vi "mkCameraMain.vi"() -> ()   [LabVIEW 2011]
uses:
  BeadTracker2.llb/GlobalVariables.vi
  BeadTracker2.llb/CmdEnum_CameraIn.ctl
  BeadTracker2.llb/CmdData_GrabParams.ctl
  BeadTracker2.llb/CmdData_NewFrame.ctl
  BeadTracker2.llb/CmdEnum_CameraFrameType.ctl
  <vilib>/vision/Image Controls.llb/IMAQ Image.ctl
  qtrk/QTrk.llb/QTrkInstance.ctl
  CameraConfig.ctl
  CameraInterface.llb/CameraInterface.ctl
  BeadTracker2.llb/GenericCameraConfigType.ctl
panel:
  in  "Test vi ref interface":bool
  in  "Camera interface":T1
  in  "Config dialog":bool
  in  "Set QTrk dll":bool
  in  "Stop":bool
  in  "Tracking test":bool
  out "# elements in Camera In":i32
  in  "EndGrab":bool
  in  "GrabIdle":bool
  in  "Init":bool
  out "Have IMAQ Session?":bool
  in  "IMAQ Session":refnum<k11>
  out "Debug Indicator:\nCurrent grab state":T2
  in  "Camera msg type":T2
  in  "Send camera msg":bool
  in  "Camera settings":T3={"Gain [1-4]"=500.0, "Offset"=2, "Mode"=75, "ROIs"=[], "ROI Size"={"X"=0, "Y"=0}, "Number of buffers"=40, "Use hardware multiple-ROI?"=TRUE, "GenericCameraConfig"={"Framerate (Hz)"=1280, "Exposure time (us)"=1024, "Image size"={"Width"=1280, "Height"=1024}}}
  # "us"
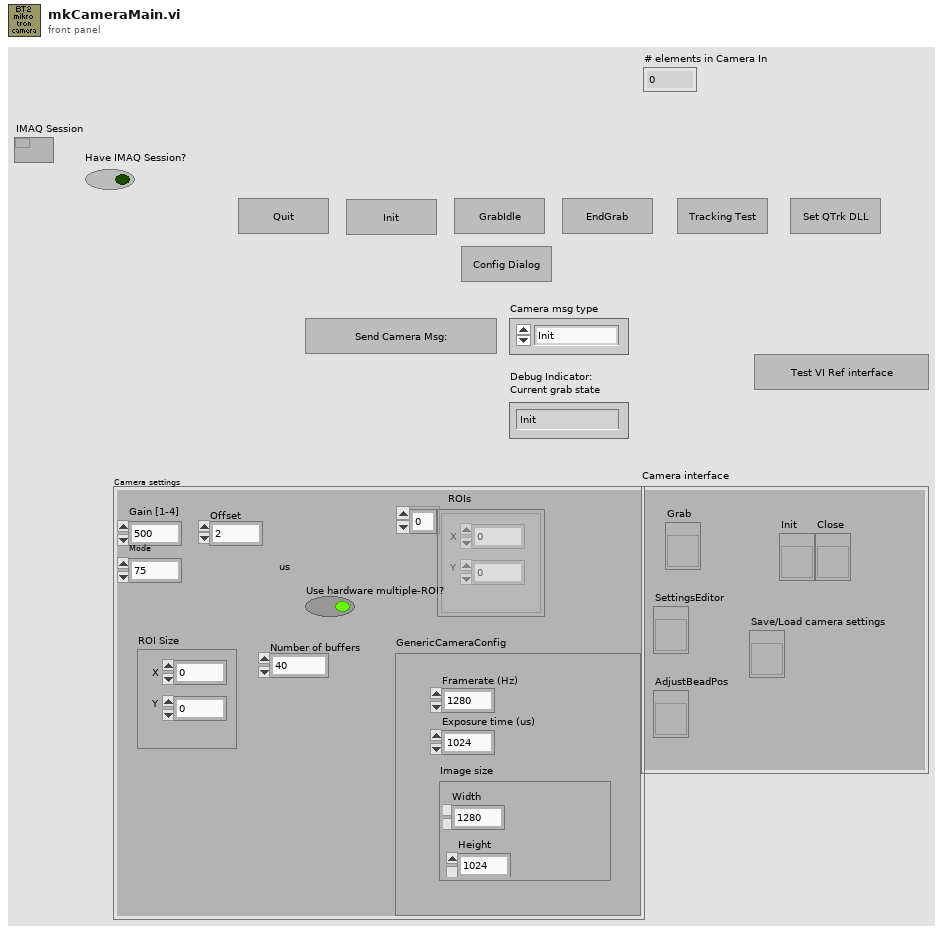
[diagram p1: front panel]
types:
  T1 = typedef "CameraInterface.ctl" = cluster{"SettingsEditor":refnum<vi>, "AdjustBeadPos":refnum<vi>, "Save/Load camera settings":refnum<vi>, "Init":refnum<vi>, "Close":refnum<vi>, "Grab":refnum<vi>}
  T2 = typedef "CmdEnum_CameraIn.ctl" = enum32{"Init", "Close", "ShowSettingsDialog", "EndGrab", "GrabZLUT", "GrabToTracker", "GrabToQueue", "AdjustROIs"}
  T3 = typedef "CameraConfig.ctl" = cluster{"Gain [1-4]":sgl, "Offset":i16, "Mode":i16, "ROIs":cluster{"X":i32, "Y":i32}[], "ROI Size":cluster{"X":i32, "Y":i32}, "Number of buffers":i32, "Use hardware multiple-ROI?":bool, "GenericCameraConfig":T4}
  T4 = typedef "GenericCameraConfigType.ctl" = cluster{"Framerate (Hz)":i32, "Exposure time (us)":i32, "Image size":cluster{"Width":i32, "Height":i32}}
  T5 = typedef "MeasureConfigType.ctl" = cluster{"Bead locations":cluster{"X":i32, "Y":i32}[], "ROI":i32, "Experiment base path":path, "Image output subdir":string, "Output mode":T6, "Traces output subdir":string, "QTrk Settings":T7, "Tracking Config":T8, "Experiment Name":string, "Program":T11, "ZLUT":sgl[][][], "Camera settings":T4, "Experiment Script":string, "Max frames in memory":i32, "Save traces as binary":bool, "Pixel Calibration Gain Image":string, "Pixel Calibration Offset Image":string, "Use pixel calibration images":bool}
  T6 = typedef "MeasureConfigOutputMode.ctl" = enum16{"None", "Track", "SaveImages"}
  T7 = typedef "QTrkSettings.ctl" = cluster{"Image width":i32, "Image height":i32, "Number of threads (CPU based)":i32, "CUDA Device":i32, "COM Background correction factor":sgl, "ZLUT MinRadius":sgl, "ZLUT Radial Coverage":sgl, "ZLUT Angular Coverage":sgl, "ZLUT ROI Coverage":sgl, "QI Iterations":i32, "QI MinRadius":sgl, "QI Radial Coverage":sgl, "QI Angular Coverage":sgl, "QI ROI Coverage":sgl, "QI Angular Step \nIteration Factor":sgl, "XCOR Profile Length":i32, "XCOR Profile Width":i32, "XCOR Iterations":i32, "Gaussian 2D Fit Iterations":i32, "Gaussian 2D Sigma (pixels)":sgl}
  T8 = typedef "TrackingConfigType.ctl" = cluster{"Number of steps":i32, "ZLUT stepsize (um)":sgl, "Z correction factor":sgl, "Start piezo Z (um)":sgl, "Pixel size (nm)":sgl, "2D Localization Type":T9, "Z Command (None)":T10}
  T9 = typedef "QTrkLocalizationType.ctl" = enum16{"Center-of-Mass", "1D Cross-Correlation", "Quadrant Interpolation", "Gaussian 2D MLE"}
  T10 = typedef "QTrkZCommandType.ctl" = enum16{"Nothing", "ComputeZ", "BuildRadialZLUT", "BuildImageZLUT", "RadialZLUT+ImageZLUT"}
  T11 = typedef "ExperimentProgramType.ctl" = cluster{"Commands":T12[], "Motor Axis accuracy conditions":T15, "Axis flags":T17}
  T12 = typedef "ExProgCommandType.ctl" = cluster{"cmd":T13, "axis":T14, "value/pos":dbl, "speed":dbl, "name":string}
  T13 = typedef "ExProgCommandEnumType.ctl" = enum16{"wait", "move", "acquire", "idle", "rmove", "when", "section", "stop"}
  T14 = typedef "MotorAxisEnum.ctl" = enum16{"no axis", "magrot", "magpos", "px", "py", "pz", "camx", "camy"}
  T15 = typedef "MotorPosType.ctl" = cluster{"Magnet Z":dbl, "Magnet rotation":dbl, "Camera":T16, "Piezo XY":T16, "Piezo Z":dbl}
  T16 = typedef "XYf.ctl" = cluster{"X":sgl, "Y":sgl}
  T17 = typedef "MotorPosFlagsType.ctl" = cluster{"Magnet Z":bool, "Magnet rotation":bool, "Camera":cluster{"X":bool, "Y":bool}, "Piezo XY":cluster{"X":bool, "Y":bool}, "Piezo Z":bool}
  T18 = typedef "QueueListType.ctl" = cluster{"Motor In":refnum<queue>, "User Interface Image View":refnum<queue>, "User Interface Camera Control":refnum<queue>, "User Interface Event Notifier":refnum<notifier>, "Initialized?":bool}
  T19 = typedef "CmdData_GrabParams.ctl" = cluster{"QTrk Instance":T20, "Output Queue":refnum<queue>}
  T20 = typedef "QTrkInstance.ctl" = cluster{"QTrk Pointer":u64}
  T21 = typedef "CmdData_NewFrame.ctl" = cluster{"Buffer Image":T22, "Frame #":i32, "Hardware ROI Index":i32, "Timestamp":dbl, "Type":T23}
  T22 = typedef "IMAQ Image.ctl" = refnum<image>
  T23 = typedef "CmdEnum_CameraFrameType.ctl" = enum16{"Full", "HardwareROI", "EndGrabMarker"}
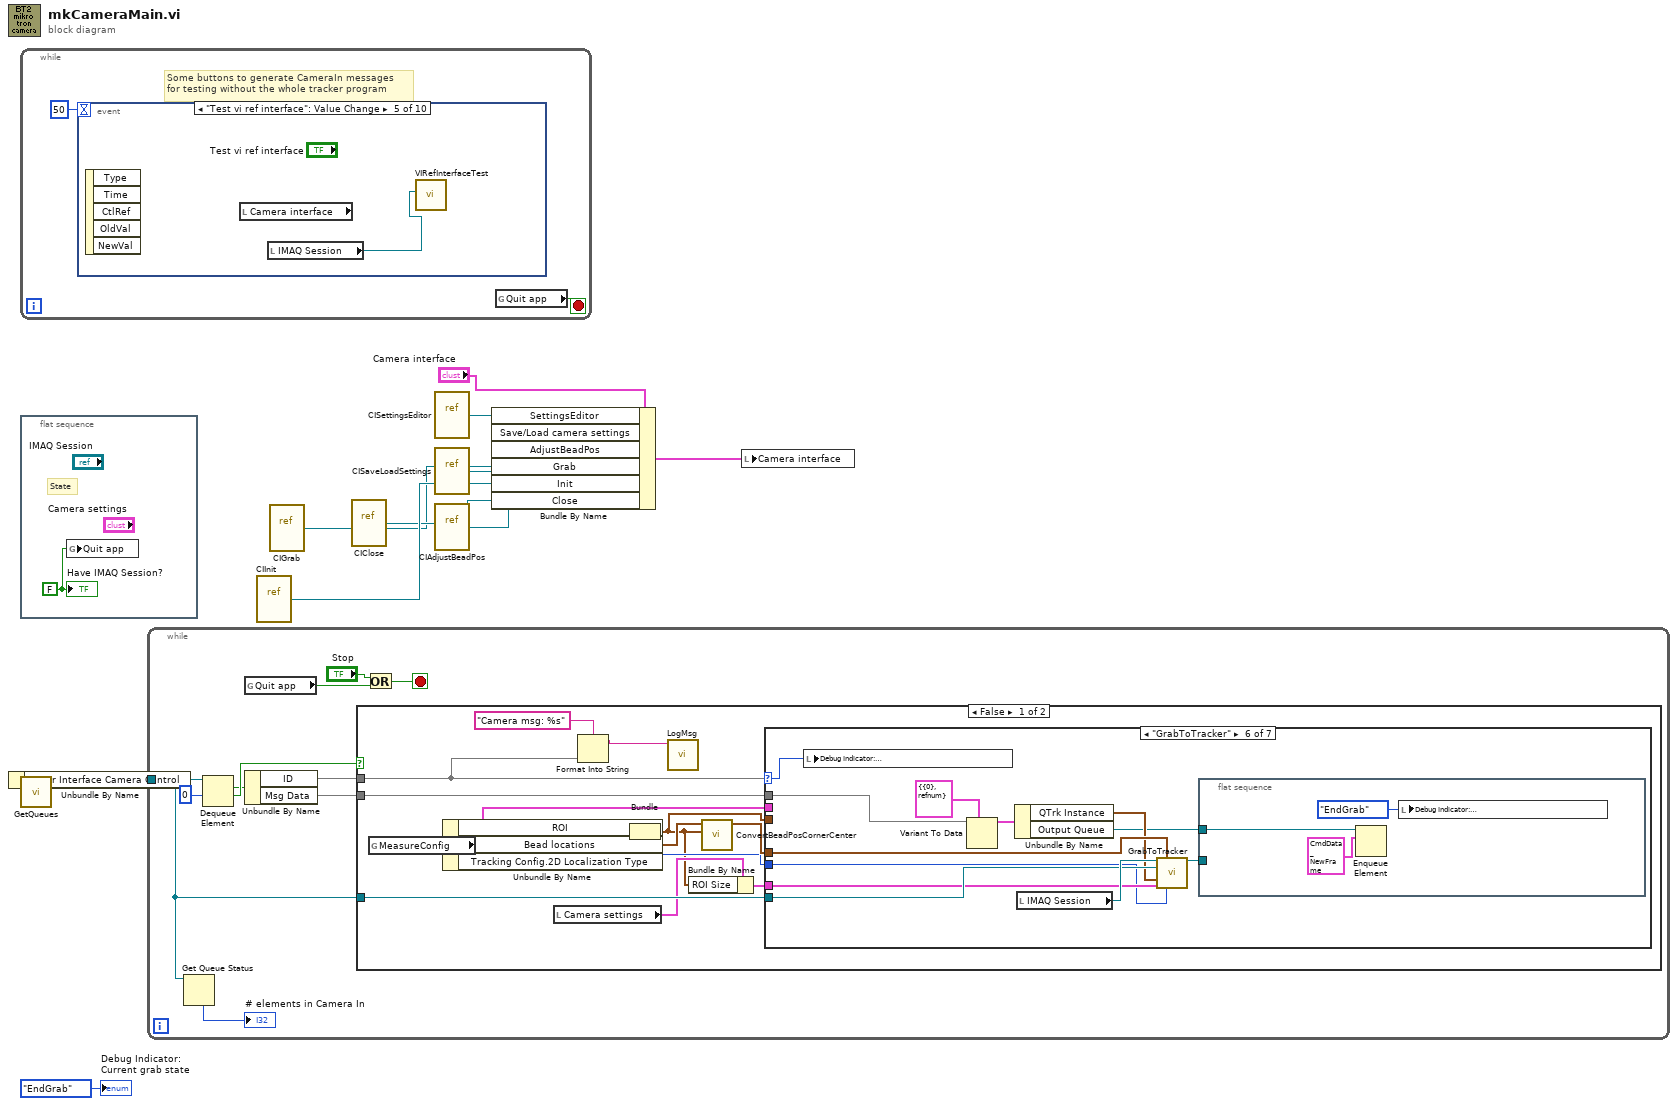
[diagram p0: block diagram]
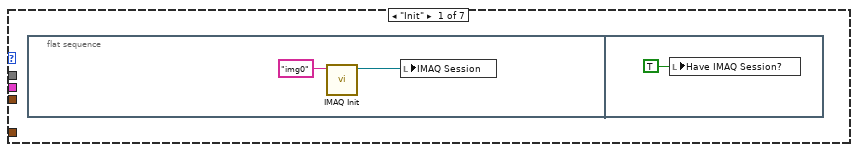
[diagram p2: hidden frame]
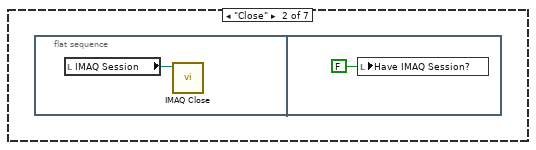
[diagram p3: hidden frame]
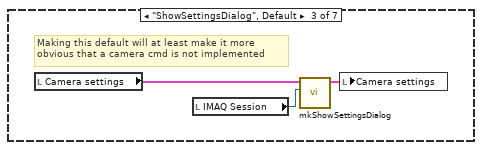
[diagram p4: hidden frame]
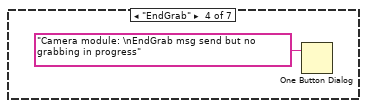
[diagram p5: hidden frame]
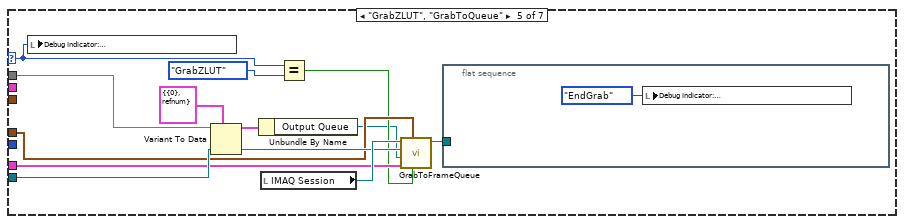
[diagram p6: hidden frame]
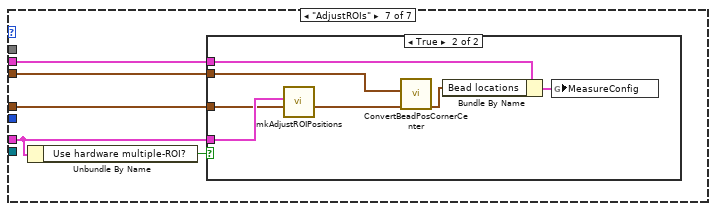
[diagram p7: hidden frame]
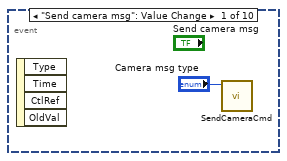
[diagram p10: hidden frame]
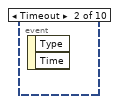
[diagram p11: hidden frame]
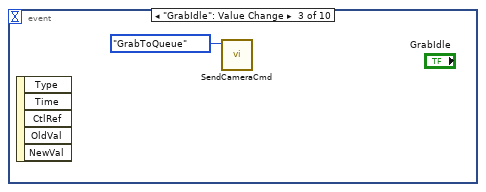
[diagram p12: hidden frame]
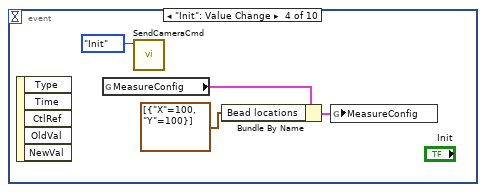
[diagram p13: hidden frame]
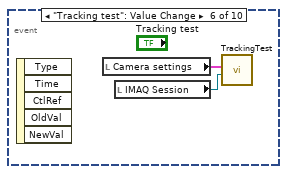
[diagram p14: hidden frame]
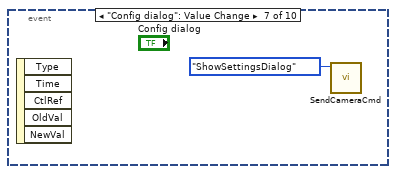
[diagram p15: hidden frame]
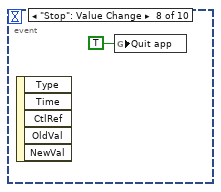
[diagram p16: hidden frame]
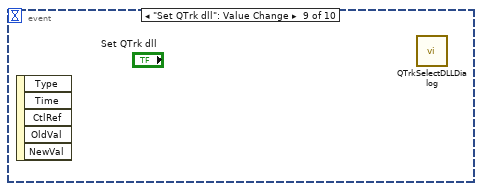
[diagram p17: hidden frame]
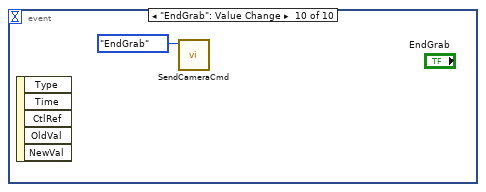
[diagram p18: hidden frame]
diagram:
  n1 = while {
    stop <- w12 stop-if-true
    # "Some buttons to generate CameraIn messages\nfor testing without the whole tracker program"
    n2 = event shown="[4] \"Test vi ref interface\": Value Change" {
      selector: _ -> [_ _ _ _ _ _ _ _ _ _]
      dyn-events: _ -> [_ _ _ _ _ _ _ _ _ _]
      timeout: 50 -> [_ _ _ _ _ _ _ _ _ _]
      event "Send camera msg": Value Change {
        n3 = event-data() -> ()  [unwired: 1 in, 4 out]
        n4 = call "SendCameraCmd.vi"("Camera cmd (SettingsDlg)"="Camera msg type") -> ()  [unwired: 11 in]
      }
      event Timeout {
        n5 = event-data() -> ()  [unwired: 1 in, 2 out]
      }
      event "GrabIdle": Value Change {
        n6 = event-data() -> ()  [unwired: 1 in, 5 out]
        n7 = call "SendCameraCmd.vi"("Camera cmd (SettingsDlg)"=CmdEnum_CameraIn."GrabToQueue" ("Camera msg type 2")) -> ()  [unwired: 11 in]
      }
      event "Init": Value Change {
        n8 = event-data() -> ()  [unwired: 1 in, 5 out]
        n9 = global read "GlobalVariables.vi" "MeasureConfig"() -> (w18:T5)
        n10 = call "SendCameraCmd.vi"("Camera cmd (SettingsDlg)"=CmdEnum_CameraIn."Init" ("Camera msg type 2")) -> ()  [unwired: 11 in]
        n11 = Bundle By Name(cluster=w18, "Bead locations"=cluster{"X":i32, "Y":i32}[] [{"X"=100, "Y"=100}]) -> (w16:T5)
        n12 = global write "GlobalVariables.vi" "MeasureConfig"(w16) -> ()
      }
      event "Test vi ref interface": Value Change {
        n13 = event-data() -> ()  [unwired: 1 in, 5 out]
        n14 = local read "Camera interface"() -> ()  [unwired: 1 out]
        n15 = local read "IMAQ Session"() -> (w20:refnum<k11>)
        n16 = call "VIRefInterfaceTest.vi"("IMAQ Session"=w20) -> ()  [unwired: 11 in]
      }
      event "Tracking test": Value Change {
        n17 = event-data() -> ()  [unwired: 1 in, 5 out]
        n18 = local read "Camera settings"() -> (w22:T3)
        n19 = local read "IMAQ Session"() -> (w21:refnum<k11>)
        n20 = call "TrackingTest.vi"("IMAQ Refnum"=w21, "Camera settings"=w22) -> ()  [unwired: 10 in]
      }
      event "Config dialog": Value Change {
        n21 = event-data() -> ()  [unwired: 1 in, 5 out]
        n22 = call "SendCameraCmd.vi"("Camera cmd (SettingsDlg)"=CmdEnum_CameraIn."ShowSettingsDialog" ("Camera msg type 2")) -> ()  [unwired: 11 in]
      }
      event "Stop": Value Change {
        n23 = event-data() -> ()  [unwired: 1 in, 5 out]
        n24 = global write "GlobalVariables.vi" "Quit app"(TRUE ("Quit app")) -> ()
      }
      event "Set QTrk dll": Value Change {
        n25 = event-data() -> ()  [unwired: 1 in, 5 out]
        n26 = call "QTrkSelectDLLDialog.vi"() -> ()  [unwired: 11 in, 1 out]
      }
      event "EndGrab": Value Change {
        n27 = event-data() -> ()  [unwired: 1 in, 5 out]
        n28 = call "SendCameraCmd.vi"("Camera cmd (SettingsDlg)"=CmdEnum_CameraIn."EndGrab" ("Camera msg type 2")) -> ()  [unwired: 11 in]
      }
    }
    n29 = global read "GlobalVariables.vi" "Quit app"() -> (w12:bool)
  }
  n30 = flat-sequence {
    frame #0 {
      w26 = FALSE ("Have IMAQ Session?")
      # "State"
      n31 = global write "GlobalVariables.vi" "Quit app"(w26) -> ()
      "Have IMAQ Session?" <- w26
    }
  }
  n32 = call "GetQueues.vi"() -> ("Queue List"=w11:T18)  [unwired: 10 in, 1 out]
  n33 = Unbundle By Name(w11) -> ("User Interface Camera Control"=w10:refnum<queue>)
  n34 = while {
    tunnel: w10 -> [w32]
    stop <- w30 stop-if-true
    n35 = Get Queue Status(queue=w32) -> (# elements in queue=→"# elements in Camera In":i32)  [unwired: 2 in, 7 out]
    n36 = Dequeue Element(queue=w32, timeout in ms (-1)=0) -> (element=w33:bool, timed out?=w35:bool)  [unwired: 1 in, 2 out]
    n37 = global read "GlobalVariables.vi" "Quit app"() -> (w29:bool)
    n38 = Unbundle By Name(w33) -> ("ID"=w34, "Msg Data"=w27)
    n39 = case shown="False" w35 {
      tunnel: w34 -> [w38 _]
      tunnel: w32 -> [w49 _]
      tunnel: w27 -> [w40 _]
      frame False {
        n40 = global read "GlobalVariables.vi" "MeasureConfig"() -> (w43:T5)
        n41 = Unbundle By Name(w43) -> ("ROI"=w47:i32, "Bead locations"=w48:cluster{"X":i32, "Y":i32}[], "Tracking Config.2D Localization Type"=w44:T9)
        n42 = local read "Camera settings"() -> (w42:T3)
        n43 = Format Into String(format string="Camera msg: %s", w38) -> (resulting string=w37:string)  [unwired: 2 in, 1 out]
        n44 = Bundle("ROI"=w47, "ROI"=w47) -> (w41:cluster{"ROI":i32, "ROI":i32})  [unwired: 1 in]
        n45 = call "LogMsg.vi"("msg"=w37) -> ()  [unwired: 11 in]
        n46 = Bundle By Name(cluster=w42, "ROI Size"=w41) -> (w45:T3)
        n47 = call "ConvertBeadPosCornerCenter.vi"("ROI Size"=w41, "Center-based bead locations"=w48) -> ("Corner-based bead pos (out)"=w46:cluster{"X":i32, "Y":i32}[])  [unwired: 8 in, 1 out]
        n48 = case shown="\"GrabToTracker\"" w38 {
          selector: w38 -> [_ _ _ _ w65 w78 _]
          tunnel: w49 -> [_ _ _ _ w69 w82 _]
          tunnel: w46 -> [_ _ _ _ w67 w81 w90]
          tunnel: w45 -> [_ _ _ _ w66 w80 w87]
          tunnel: w44 -> [_ _ _ _ _ w79 _]
          tunnel: w43 -> [_ _ _ _ _ _ w88]
          tunnel: w41 -> [_ _ _ _ _ _ w89]
          tunnel: w40 -> [_ _ _ _ w62 w76 _]
          frame "Init" {
            n49 = flat-sequence {
              frame #0 {
                n50 = call <vilib>:"IMAQ Init.vi"("Interface Name"="img0") -> ("IMAQ Session Out"=w50:refnum<k11>)  [unwired: 9 in, 1 out]
                n51 = local write "IMAQ Session"(w50) -> ()
              }
              frame #1 {
                n52 = local write "Have IMAQ Session?"(TRUE ("Have IMAQ Session?")) -> ()
              }
            }
          }
          frame "Close" {
            n53 = flat-sequence {
              frame #0 {
                n54 = local read "IMAQ Session"() -> (w53:refnum<k11>)
                n55 = call <vilib>:"IMAQ Close.vi"("IMAQ Session In"=w53) -> ()  [unwired: 10 in, 1 out]
              }
              frame #1 {
                n56 = local write "Have IMAQ Session?"(FALSE ("Have IMAQ Session?")) -> ()
              }
            }
          }
          frame "ShowSettingsDialog", Default {
            # "Making this default will at least make it more \nobvious that a camera cmd is not implemented"
            n57 = local read "Camera settings"() -> (w57:T3)
            n58 = local read "IMAQ Session"() -> (w56:refnum<k11>)
            n59 = call "mkShowSettingsDialog.vi"("IMAQ Refnum"=w56, "Camera (in)"=w57) -> ("Camera (out)"=w55:T3)  [unwired: 9 in]
            n60 = local write "Camera settings"(w55) -> ()
          }
          frame "EndGrab" {
            n61 = One Button Dialog(message="Camera module: \nEndGrab msg send but no grabbing in progress") -> ()  [unwired: 1 in, 1 out]
          }
          frame "GrabZLUT", "GrabToQueue" {
            n62 = local write "Debug Indicator:\nCurrent grab state"(w65) -> ()
            n63 = Variant To Data(type=T19 {"QTrk Instance"={"QTrk Pointer"=0}, "Output Queue"=refnum} ("GrabToTrackerParameters"), Variant=w62) -> (data=w60:T19)  [unwired: 1 in, 1 out]
            n64 = Unbundle By Name(w60) -> ("Output Queue"=w59:refnum<queue>)
            n65 = local read "IMAQ Session"() -> (w70:refnum<k11>)
            n66 = Equal?(x=w65, y=CmdEnum_CameraIn."GrabZLUT" ("ID")) -> (x = y?=w63:bool)
            n67 = call "GrabToFrameQueue.vi"("Building ZLUT?"=w63, "ROI corner pos"=w67, "Camera settings"=w66, "Camera Out"=w59, "Camera In"=w69, "IMAQ Refnum"=w70) -> ("IMAQ Session Out"=w64:refnum<k11>)  [unwired: 5 in]
            n68 = flat-sequence {
              tunnel: w64 -> [_]
              frame #0 {
                n69 = local write "Debug Indicator:\nCurrent grab state"(CmdEnum_CameraIn."EndGrab" ("Current grab state")) -> ()
              }
            }
          }
          frame "GrabToTracker" {
            n70 = local write "Debug Indicator:\nCurrent grab state"(w78) -> ()
            n71 = Variant To Data(type=T19 {"QTrk Instance"={"QTrk Pointer"=0}, "Output Queue"=refnum} ("GrabToTrackerParameters"), Variant=w76) -> (data=w74:T19)  [unwired: 1 in, 1 out]
            n72 = Unbundle By Name(w74) -> ("QTrk Instance"=w73:T20, "Output Queue"=w72:refnum<queue>)
            n73 = local read "IMAQ Session"() -> (w83:refnum<k11>)
            n74 = call "GrabToTracker.vi"("IMAQ Refnum"=w83, "ROI corner pos"=w81, "Camera In"=w82, "QTrk Instance"=w73, "Camera settings"=w80, "2D Localization Type (COM)"=w79) -> ("IMAQ Session Out"=w77:refnum<k11>)  [unwired: 9 in]
            n75 = flat-sequence {
              tunnel: w77 -> [_]
              tunnel: w72 -> [w85]
              frame #0 {
                n76 = Enqueue Element(queue=w85, element=T21 {"Buffer Image"=refnum, "Frame #"=0, "Hardware ROI Index"=0, "Timestamp"=0.0, "Type"=enum."EndGrabMarker"}) -> ()  [unwired: 2 in, 3 out]
                n77 = local write "Debug Indicator:\nCurrent grab state"(CmdEnum_CameraIn."EndGrab" ("Debug Indicator:\nCurrent grab state")) -> ()
              }
            }
          }
          frame "AdjustROIs" {
            n78 = Unbundle By Name(w87) -> ("Use hardware multiple-ROI?"=w91:bool)
            n79 = case shown="True" w91 {
              tunnel: w87 -> [_ w98]
              tunnel: w90 -> [_ w97]
              tunnel: w89 -> [_ w96]
              tunnel: w88 -> [_ w94]
              frame False {
              }
              frame True {
                n80 = call "mkAdjustROIPositions.vi"("Corner-based bead pos"=w97, "Camera settings"=w98) -> ("Adjusted bead pos (out)"=w95:cluster{"X":i32, "Y":i32}[])  [unwired: 9 in]
                n81 = call "ConvertBeadPosCornerCenter.vi"("Corner-based bead locations"=w95, "ROI Size"=w96) -> ("Center-based bead pos (out)"=w93:cluster{"X":i32, "Y":i32}[])  [unwired: 8 in, 1 out]
                n82 = Bundle By Name(cluster=w94, "Bead locations"=w93) -> (w92:T5)
                n83 = global write "GlobalVariables.vi" "MeasureConfig"(w92) -> ()
              }
            }
          }
        }
      }
      frame True {
      }
    }
    n84 = Or(x="Stop", y=w29) -> (x .or. y?=w30:bool)
  }
  n85 = vi-ref "CIInit.vi"() -> (w3:refnum<vi>)
  n86 = vi-ref "CIGrab.vi"() -> (w1:refnum<vi>)
  n87 = vi-ref "CIClose.vi"() -> (w2:refnum<vi>)
  n88 = vi-ref "CISettingsEditor.vi"() -> (w4:refnum<vi>)
  n89 = vi-ref "CISaveLoadSettings.vi"() -> (w5:refnum<vi>)
  n90 = vi-ref "CIAdjustBeadPos.vi"() -> (w6:refnum<vi>)
  n91 = Bundle By Name(cluster="Camera interface", "SettingsEditor"=w4, "Save/Load camera settings"=w5, "AdjustBeadPos"=w6, "Grab"=w1, "Init"=w3, "Close"=w2) -> (w7:T1)
  n92 = local write "Camera interface"(w7) -> ()
  "Debug Indicator:\nCurrent grab state" <- CmdEnum_CameraIn."EndGrab" ("Current grab state")
